vi "Apogee_Global.vi"() -> ()   [LabVIEW 2015]
uses:
  SI_Client_Subvis/CameraStates.ctl
panel:
  in  "Camera State":T1
  out "Apogee Online":bool
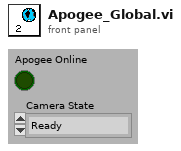
[diagram p1: front panel]
types:
  T1 = typedef "CameraStates.ctl" = enum16{"Ready", "Exposing", "Error"}
diagram:
